vi "Compare Key.vi"(1 "keyB in":cluster{"(g or v) + h":dbl, "g or v":dbl}, 2 "keyA in":cluster{"(g or v) + h":dbl, "g or v":dbl}) -> (0 "keyA > keyB":bool)   [LabVIEW 2017, in "NI_Robotics_AnytimeDStar.lvclass"]
uses:
  <vilib>/robotics/Navigation/Anytime D Star/NI_Robotics_AnytimeDStar.lvclass
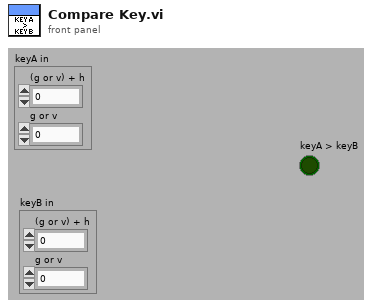
[diagram p1: front panel]
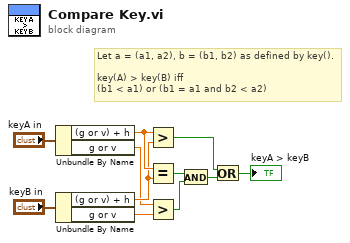
[diagram p0: block diagram]
diagram:
  # "Let a = (a1, a2), b = (b1, b2) as defined by key().\n\nkey(A) > key(B) iff\n(b1 < a1) or (b1 = a1 and b2 < a2)"
  n1 = Unbundle By Name("keyA in") -> ("(g or v) + h"=w7:dbl, "g or v"=w3:dbl)
  n2 = Unbundle By Name("keyB in") -> ("(g or v) + h"=w6:dbl, "g or v"=w2:dbl)
  n3 = Greater?(x=w7, y=w6) -> (0:w8:bool)
  n4 = Equal?(x=w7, y=w6) -> (x = y?=w5:bool)
  n5 = Greater?(x=w3, y=w2) -> (0:w1:bool)
  n6 = And(x=w5, y=w1) -> (x .and. y?=w4:bool)
  n7 = Or(x=w8, y=w4) -> (x .or. y?=→"keyA > keyB":bool)
